vi "SetDC.vi"(3 "error in (no error)":errorcluster, 4 "DC(=DTR) state":i16 min=0 max=1 step=1, 5 "VISA resource":refnum<visa-resource-name>="COM1") -> (0 "error out":errorcluster, 2 "dup VISA resource":refnum<visa-resource-name>="COM1")   [LabVIEW 2023]
doc: "Controls state of data signal\nto AVS-47B"
panel:
  # "SetDC.vi"
  # "This VI controls the state (1 or 0)  of the DC (Data from Computer) Picobus output  line (DTR handshake of COM port)."
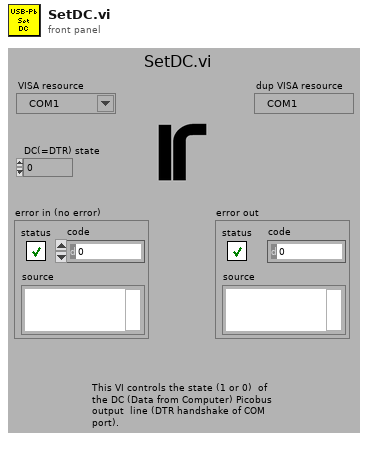
[diagram p1: front panel]
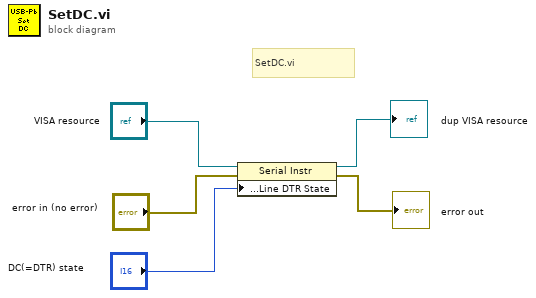
[diagram p0: block diagram]
diagram:
  # "SetDC.vi"
  n1 = property class="Serial Instr"(reference="VISA resource", error in="error in (no error)", "Serial Settings:Modem Line Settings:Line DTR State"="DC(=DTR) state") -> (reference out=→"dup VISA resource":refnum<visa-resource-name>, error out=→"error out":errorcluster)
